vi "Read_Data.vi"(8 "error in":errorcluster caption="entrée d'erreur") -> (0 "error out":errorcluster caption="sortie d'erreur", 1 "Waveform Graph 2":waveform(dbl)[](graph)=[{"t0"=timestamp(0 s since 1904-01-01), "dt"=1e-05, "Y"=array[75000 elements]}, {"t0"=timestamp(0 s since 1904-01-01), "dt"=1e-05, "Y"=array[75000 elements]}, {"t0"=timestamp(0 s since 1904-01-01), "dt"=1e-05, "Y"=array[75000 elements]}], 2 "Waveform Graph":waveform(dbl)[](graph)=[{"t0"=timestamp(0 s since 1904-01-01), "dt"=1e-05, "Y"=array[75000 elements]}, {"t0"=timestamp(0 s since 1904-01-01), "dt"=1e-05, "Y"=array[75000 elements]}, {"t0"=timestamp(0 s since 1904-01-01), "dt"=1e-05, "Y"=array[75000 elements]}, {"t0"=timestamp(0 s since 1904-01-01), "dt"=1e-05, "Y"=array[75000 elements]}], 3 "DO WF OUT":digitalwaveform(graph))   [LabVIEW 2026]
uses:
  FGV/TypeDef_FGV.ctl
  <vilib>/Waveform/DWDTOps.llb/DWDT Boolean Array to Digital.vi
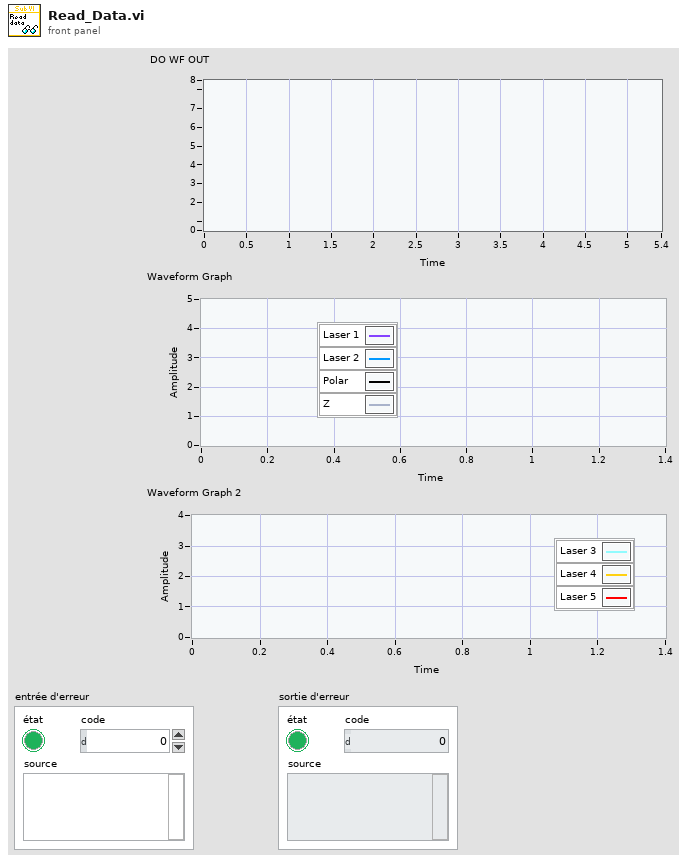
[diagram p1: front panel]
types:
  T1 = typedef "TypeDef_FGV.ctl" = enum16{"Initialize", "Write", "Read", "Read_File", "Write_to_File"}
  T2 = enum16{"big-endian, network order", "native, host order", "little-endian"}
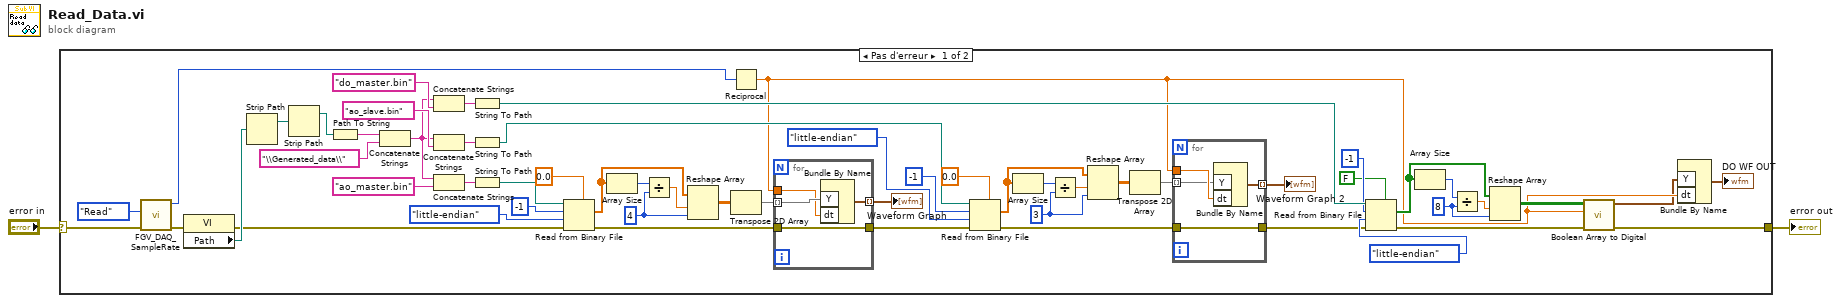
[diagram p0: block diagram]
diagram:
  n1 = case shown="Pas d'erreur" "error in" {
    selector: "error in" -> [w23 w68]
    tunnel: [w3 w68] -> w1
    frame No Error {
      w30 = u8 8 ("Nber of columns to read")
      w41 = u8 3 ("Nber of columns to read")
      w50 = u8 4 ("Nber of columns to read")
      n2 = call "FGV_DAQ_SampleRate.vi"("error in"=w23, "Action"=TypeDef_FGV."Read") -> ("error out"=w21:errorcluster, "Sample rate OUT"=w20:u32)  [unwired: 8 in]
      n3 = property class="VI"(error in=w21) -> (error out=w55:errorcluster, "Path"=w58:path)  [unwired: 1 in, 1 out]
      n4 = Strip Path(path=w58) -> (stripped path=w57:path)  [unwired: 1 out]
      n5 = Strip Path(path=w57) -> (stripped path=w56:path)  [unwired: 1 out]
      n6 = Path To String(path=w56) -> (string=w59:string)
      n7 = Concatenate Strings(w59, "\\Generated_data\\" ("Python_file")) -> (w25:string)
      n8 = Concatenate Strings(w25, "do_master.bin" ("File_to_read")) -> (w35:string)
      n9 = Concatenate Strings(w25, "ao_slave.bin" ("File_to_read")) -> (w36:string)
      n10 = Concatenate Strings(w25, "ao_master.bin" ("File_to_read")) -> (w54:string)
      n11 = String To Path(string=w35) -> (path=w34:path)
      n12 = String To Path(string=w36) -> (path=w37:path)
      n13 = String To Path(string=w54) -> (path=w53:path)
      n14 = Read from Binary File(5:0.0, 8:w55, 9:T2."little-endian" ("ordre des octets (0 : big-Endian, network order)"), 10:-1 ("nombre (1)"), 11:w53) -> (0:w7:errorcluster, 2:w24:dbl[])  [unwired: 1 in, 2 out]
      n15 = Array Size(array=w24) -> (size(s)=w49:i32)
      n16 = Divide(x=w49, y=w50) -> (x/y=w48:dbl)
      n17 = Reshape Array(w24, w48, w50) -> (w14:dbl[][])
      n18 = Reciprocal(x=w20) -> (1/x=w11:dbl)
      n19 = Transpose 2D Array(2D array=w14) -> (transposed array=w13:dbl[][])
      n20 = for {
        tunnel: w13 -> [w67] mode=indexing
        tunnel: w11 -> [w66]
        tunnel: [w65] -> w19 mode=indexing
        tunnel: [w64] -> w8
        tunnel: w7 -> [w64]
        n21 = Bundle By Name("Y"=w67, "dt"=w66) -> (w65:waveform(dbl))  [unwired: 1 in]
      }
      "Waveform Graph" <- w19
      n22 = Read from Binary File(5:0.0, 8:w8, 9:T2."little-endian" ("ordre des octets (0 : big-Endian, network order)"), 10:-1 ("nombre (1)"), 11:w37) -> (0:w6:errorcluster, 2:w39:dbl[])  [unwired: 1 in, 2 out]
      n23 = Array Size(array=w39) -> (size(s)=w42:i32)
      n24 = Divide(x=w42, y=w41) -> (x/y=w43:dbl)
      n25 = Reshape Array(w39, w43, w41) -> (w18:dbl[][])
      n26 = Transpose 2D Array(2D array=w18) -> (transposed array=w12:dbl[][])
      n27 = for {
        tunnel: w11 -> [w63]
        tunnel: [w62] -> w17 mode=indexing
        tunnel: w12 -> [w61] mode=indexing
        tunnel: w6 -> [w60]
        tunnel: [w60] -> w5
        n28 = Bundle By Name("Y"=w61, "dt"=w63) -> (w62:waveform(dbl))  [unwired: 1 in]
      }
      "Waveform Graph 2" <- w17
      n29 = Read from Binary File(5:FALSE, 8:w5, 9:T2."little-endian" ("ordre des octets (0 : big-Endian, network order)"), 10:-1 ("nombre (1)"), 11:w34) -> (0:w4:errorcluster, 2:w32:bool[])  [unwired: 1 in, 2 out]
      n30 = Array Size(array=w32) -> (size(s)=w29:i32)
      n31 = Divide(x=w29, y=w30) -> (x/y=w28:dbl)
      n32 = Reshape Array(w32, w28, w30) -> (w15:bool[][])
      n33 = call-poly <vilib>:"Boolean Array to Digital.vi"("error in (no error)"=w4, "sample rate"=w11, "boolean array"=w15) -> ("error out"=w3:errorcluster, "digital waveform"=w10:digitalwaveform)  [unwired: 7 in]
      n34 = Bundle By Name ("Construire une waveform")("Y"=w10, "dt"=w11) -> (→"DO WF OUT":digitalwaveform)  [unwired: 1 in]
    }
    frame Error {
    }
  }
  "error out" <- w1
